vi "DigitalOutput-Start.vi"(3 "error in (no error)":errorcluster, 4 "OutputRequest\nuser event refnum":T1, 5 "Configuration":T2={"Output Lines"=["6289/port0/line1", "6289/port0/line2", "6289/port0/line3", "6289/port0/line4", "6289/port0/line5", "6289/port0/line6", "6289/port0/line7"], "DO timestamp lines"=["6289/port0/line1", "6289/port0/line2", "6289/port0/line3", "6289/port0/line4", "6289/port0/line5", "6289/port0/line6", "6289/port0/line7"], "Timestamp lines"=[]}) -> (0 "error out":errorcluster)   [LabVIEW 2015]
uses:
  DigitalOutput-Configuration.ctl
  Typedefs/OutputRequest refnum.ctl
  Typedefs/OutputRequest.ctl
panel:
  # "Timestamp lines must be on same device as its corresponding DO line"
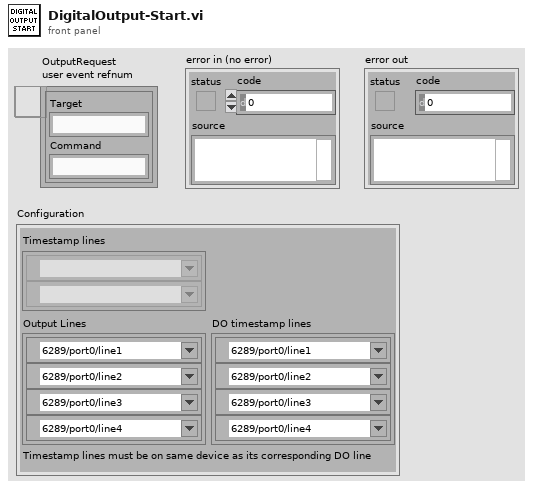
[diagram p1: front panel]
types:
  T1 = typedef "OutputRequest refnum.ctl" = refnum<user-event>
  T2 = typedef "DigitalOutput-Configuration.ctl" = cluster{"Output Lines":tag[], "DO timestamp lines":tag[], "Timestamp lines":tag[]}
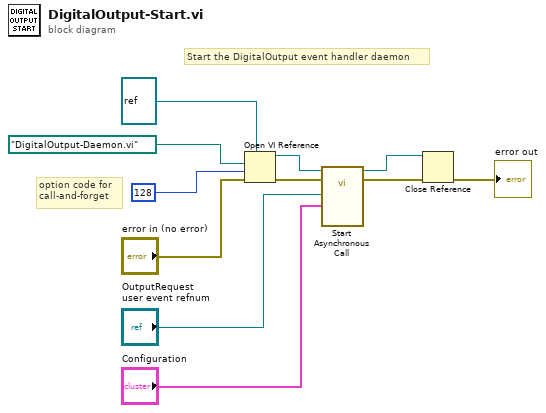
[diagram p0: block diagram]
diagram:
  # "option code for\ncall-and-forget"
  # "Start the DigitalOutput event handler daemon"
  n1 = Open VI Reference(type specifier VI Refnum (for type only)=refnum<vi> refnum, vi path=path "DigitalOutput-Daemon.vi", options=128, error in (no error)="error in (no error)") -> (vi reference=w10:refnum<vi>, error out=w11:errorcluster)  [unwired: 2 in]
  n2 = call-by-ref "Start Asynchronous Call"(reference=w10, error in=w11, "Configuration"="Configuration", "OutputRequest\nuser event refnum"="OutputRequest\nuser event refnum") -> (reference out=w6:refnum<vi>, error out=w7:errorcluster)  [unwired: 3 in]
  n3 = Close Reference(reference=w6, error in (no error)=w7) -> (error out=→"error out":errorcluster)
